vi "Init.vi"(6 "InitFlags":T1 items=["NONE"=0, "SDL_INIT_AUDIO"=16, "SDL_INIT_VIDEO"=32, "SDL_INIT_JOYSTICK"=512, "SDL_INIT_HAPTIC"=4096, "SDL_INIT_GAMEPAD"=8192, "SDL_INIT_EVENTS"=16384, "SDL_INIT_SENSOR"=32768, "SDL_INIT_CAMER"=65536], 8 "No Error":errorcluster) -> (0 "error out":errorcluster)   [LabVIEW 2026, in "SDL3.lvlib" / "Init.lvlib"]
doc: "<B>Summary</B>\nInitialize the SDL library.\n\n<B>Remarks</B>\n<B>SDL_Init()</B> simply forwards to calling <B>SDL_InitSubSystem()</B>. Therefore, the two may be used interchangeably. Though for readability of your code <B>SDL_InitSubSystem()</B> might be preferred.\n\nThe file I/O (for example: <B>SDL_IOFromFile</B>) and threading (<B>SDL_CreateThread</B>) subsystems are initialized by default. Message boxes (<B>SDL_ShowSimpleMessageBox</B>) also attempt to work without initializing the video subsystem, in hopes of being useful in showing an error dialog when <B>SDL_Init</B> fails. You must specifically initialize other subsystems if you use them in your application.\n\nLogging (such as <B>SDL_Log</B>) works without initialization, too.\n\nflags may be any of the following OR'd together:\n\n- <B>SDL_INIT_AUDIO</B>: audio subsystem; automatically initializes the events subsystem\n- <B>SDL_INIT_VIDEO</B>: video subsystem; automatically initializes the events subsystem\n- <B>SDL_INIT_JOYSTICK</B>: joystick subsystem; automatically initializes the events subsystem\n- <B>SDL_INIT_HAPTIC</B>: haptic (force feedback) subsystem\n- <B>SDL_INIT_GAMEPAD</B>: gamepad subsystem; automatically initializes the joystick subsystem\n- <B>SDL_INIT_EVENTS</B>: events subsystem\n- <B>SDL_INIT_SENSOR</B>: sensor subsystem; automatically initializes the events subsystem\n- <B>SDL_INIT_CAMERA</B>: camera subsystem; automatically initializes the events subsystem\nSubsystem initialization is ref-counted, you must call <B>SDL_QuitSubSystem()</B> for each <B>SDL_InitSubSystem()</B> to correctly shutdown a subsystem manually (or call <B>SDL_Quit()</B> to force shutdown). If a subsystem is already loaded then this call will increase the ref-count and return.\n\nConsider reporting some basic metadata about your application before calling <B>SDL_Init</B>, using either <B>SDL_SetAppMetadata()</B> or <B>SDL_SetAppMetadataProperty()</B>."
uses:
  Init.lvlib
  InitFlags--ring.ctl
  <vilib>/Utility/error.llb/Error Cluster From Error Code.vi
  Error/Error.lvlib
  Lib/SDL3.dll
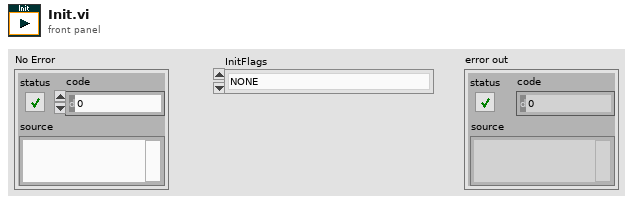
[diagram p1: front panel]
types:
  T1 = typedef "SDL3.lvlib/Init.lvlib/InitFlags--ring.ctl" = u32
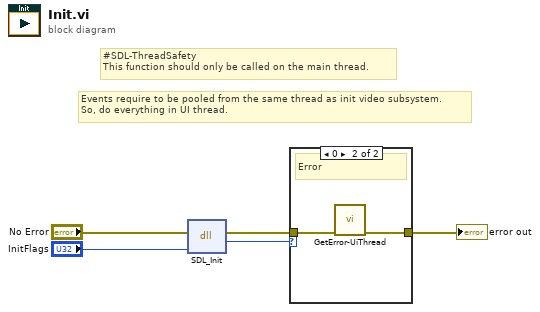
[diagram p0: block diagram]
diagram:
  # "#SDL-ThreadSafety\nThis function should only be called on the main thread."
  # "Events require to be pooled from the same thread as init video subsystem.\nSo, do everything in UI thread."
  n1 = dll-call lib="C:/Users/saukko/Dev/LV-SDL3/Sources/SDL3/Lib/SDL3.*" fn="SDL_Init"(error in="No Error", "flags"="InitFlags") -> (error out=w1:errorcluster, "return type"=w2:i32)  [unwired: 3 in, 1 out]
  n2 = case shown="0" w2 {
    tunnel: w1 -> [w6 w8]
    tunnel: [w6 w7] -> w4
    frame Default {
      # "Ok"
    }
    frame 0 {
      # "Error"
      n3 = call "GetError-UiThread.vi"("No Error"=w8) -> ("error out"=w7:errorcluster)  [unwired: 10 in]
    }
  }
  "error out" <- w4
